vi "Configure PFI Channels.vi"(8 "Error In":errorcluster, 10 "channel list (all:\"\")":string="PFI24,PFI25", 11 "instrument handle":refnum<k15>) -> (0 "Error Out":errorcluster)   [LabVIEW 2013]
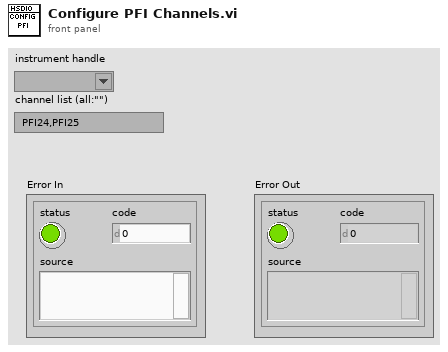
[diagram p1: front panel]
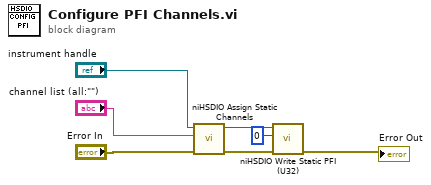
[diagram p0: block diagram]
diagram:
  n1 = call <instrlib>:"niHSDIO Assign Static Channels.vi"("error in (no error)"="Error In", "channel list (all:\"\")"="channel list (all:\"\")", "instrument handle"="instrument handle") -> ("error out"=w5:errorcluster, "instrument handle out"=w4:refnum<k15>)  [unwired: 7 in]
  n2 = call <instrlib>:"niHSDIO Write Static PFI (U32).vi"("error in (no error)"=w5, "write data (0x0000)"=u32 0, "instrument handle"=w4) -> ("error out"=→"Error Out":errorcluster)  [unwired: 7 in, 1 out]
